vi "Write Virtual Camera Configuration.vi"(8 "error in (no error)":errorcluster, 10 "Virtual Camera Configuration":T1, 11 "Virtual Camera in":refnum<class "Virtual Camera.lvclass">) -> (0 "error out":errorcluster, 3 "Virtual Camera out":refnum<class "Virtual Camera.lvclass">)   [LabVIEW 2018, in "Virtual Camera.lvlib" / "Virtual Camera.lvclass"]
uses:
  Virtual Camera.lvclass
  Resources/Type Defs/Virtual Camera Configuration.ctl
  Resources/Type Defs/Camera Type.ctl
  Virtual Camera.lvclass/Virtual Camera.ctl
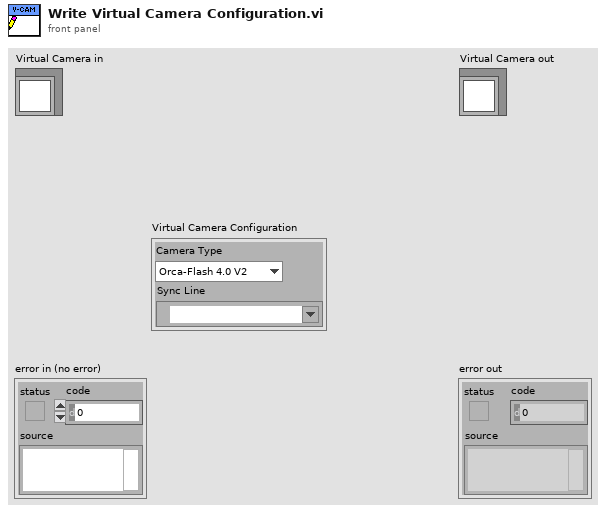
[diagram p1: front panel]
types:
  T1 = typedef "Virtual Camera Configuration.ctl" = cluster{"Camera Type":T2, "Sync Line":tag}
  T2 = typedef "Camera Type.ctl" = enum16{"Orca-Flash 4.0 V2"}
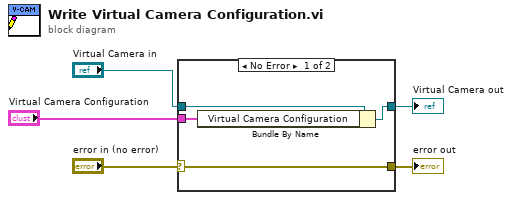
[diagram p0: block diagram]
diagram:
  n1 = case shown="No Error" "error in (no error)" {
    selector: "error in (no error)" -> [w9 w10]
    tunnel: [w9 w10] -> w4
    tunnel: [w7 w11] -> w2
    tunnel: "Virtual Camera in" -> [w8 w11]
    tunnel: "Virtual Camera Configuration" -> [w6 _]
    frame No Error {
      n2 = Bundle By Name(cluster=w8, "Virtual Camera Configuration"=w6) -> (w7:refnum<class "Virtual Camera.lvclass">)
    }
    frame Error {
    }
  }
  "error out" <- w4
  "Virtual Camera out" <- w2
